vi "Parse Geometric Element with Fast Tree.vi"(8 "error in":errorcluster, 10 "Node":T1, 11 "ParseGDSII in":refnum<class "ParseGDSII.lvclass">) -> (0 "error out":errorcluster, 2 "Geometric Objects":refnum<class "Geometric.lvclass">[](array[class]), 3 "ParseGDSII out":refnum<class "ParseGDSII.lvclass">)   [LabVIEW 2019, in "ParseGDSII.lvclass"]
uses:
  ParseGDSII.lvclass
  Elements/Geometric.lvclass
  ParseGDSII.lvclass/ParseGDSII.ctl
  Fast Tree/Fast Tree.lvclass
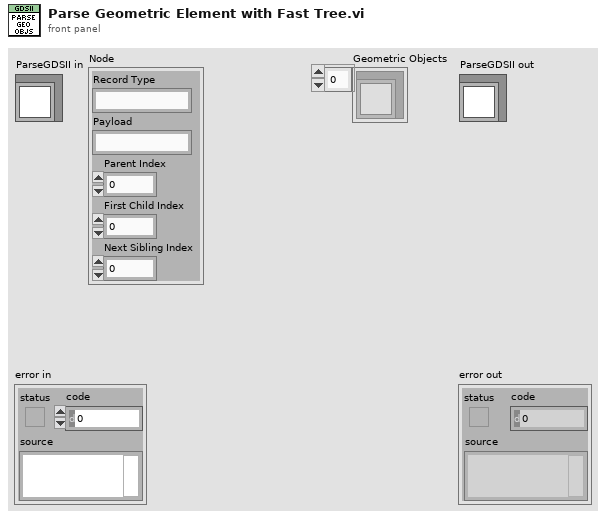
[diagram p1: front panel]
types:
  T1 = cluster{"Record Type":string, "Payload":string, "Parent Index":i32, "First Child Index":i32, "Next Sibling Index":i32}
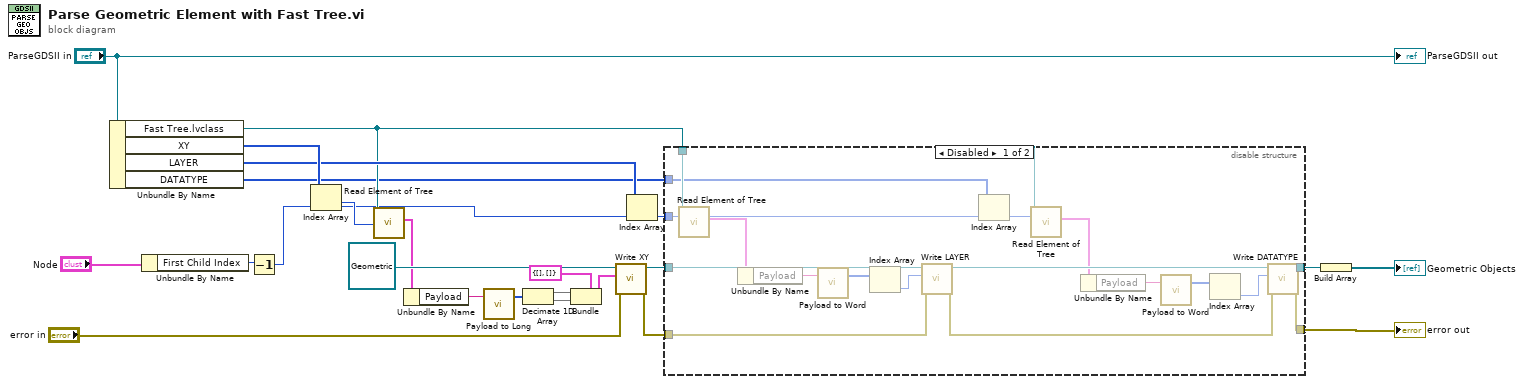
[diagram p0: block diagram]
diagram:
  n1 = Unbundle By Name("ParseGDSII in") -> ("Fast Tree.lvclass"=w3:refnum<class "Fast Tree.lvclass">, "XY"=w12:i32[], "LAYER"=w6:i32[], "DATATYPE"=w2:i32[])
  n2 = Unbundle By Name("Node") -> ("First Child Index"=w10:i32)
  n3 = Decrement(x=w10) -> (x-1=w1:i32)
  n4 = Index Array(array=w12, index=w1) -> (element=w9:i32)
  n5 = call "Read Element of Tree.vi"("index"=w9, "Fast Tree in"=w3) -> ("Node"=w8:T1)  [unwired: 7 in, 2 out]
  n6 = Unbundle By Name(w8) -> ("Payload"=w15:string)
  n7 = call "Payload to Long.vi"("Payload"=w15) -> ("Long"=w18:i32[])  [unwired: 2 in]
  n8 = Decimate 1D Array(w18) -> (w21:i32[], w20:i32[])
  n9 = Bundle(cluster=cluster{"X":i32[], "Y":i32[]} {"X"=[], "Y"=[]} ("XY"), "X"=w21, "Y"=w20) -> (w17:cluster{"X":i32[], "Y":i32[]})
  n10 = call-dynamic "Write XY.vi"("error in (no error)"="error in", "XY"=w17, "Element in"=refnum<class "Geometric.lvclass"> refnum ("Geometric")) -> ("error out"=w4:errorcluster, "Element out"=w23:refnum<class "Geometric.lvclass">)  [unwired: 7 in]
  n11 = Index Array(array=w6, index=w1) -> (element=w5:i32)
  n12 = disable-structure shown="Disabled" {
    disable-tunnel: w23 -> [w42 w45]
    disable-tunnel: [w39 w45] -> w22
    disable-tunnel: [w34 w44] -> w13
    disable-tunnel: w5 -> [w33 _]
    disable-tunnel: w4 -> [w31 w44]
    disable-tunnel: w3 -> [w28 _]
    disable-tunnel: w2 -> [w27 _]
    disable-tunnel: w1 -> [w26 _]
    frame Disabled {
      n13 = call "Read Element of Tree.vi"("index"=w33, "Fast Tree in"=w28) -> ("Node"=w32:T1)  [unwired: 7 in, 2 out]
      n14 = Unbundle By Name(w32) -> ("Payload"=w38:string)
      n15 = call "Payload to Word.vi"("Payload"=w38) -> ("Word"=w37:i16[])  [unwired: 2 in]
      n16 = Index Array(array=w37) -> (element=w43:i16)  [unwired: 1 in]
      n17 = call-dynamic "Write LAYER.vi"("error in (no error)"=w31, "LAYER"=w43, "Geometric in"=w42) -> ("error out"=w30:errorcluster, "Geometric out"=w40:refnum<class "Geometric.lvclass">)  [unwired: 7 in]
      n18 = Index Array(array=w27, index=w26) -> (element=w29:i32)
      n19 = call "Read Element of Tree.vi"("index"=w29, "Fast Tree in"=w28) -> ("Node"=w25:T1)  [unwired: 7 in, 2 out]
      n20 = Unbundle By Name(w25) -> ("Payload"=w36:string)
      n21 = call "Payload to Word.vi"("Payload"=w36) -> ("Word"=w35:i16[])  [unwired: 2 in]
      n22 = Index Array(array=w35) -> (element=w41:i16)  [unwired: 1 in]
      n23 = call-dynamic "Write DATATYPE.vi"("error in (no error)"=w30, "DATATYPE"=w41, "Geometric in"=w40) -> ("error out"=w34:errorcluster, "Geometric out"=w39:refnum<class "Geometric.lvclass">)  [unwired: 7 in]
    }
    frame Enabled {
    }
  }
  "error out" <- w13
  n24 = Build Array(w22) -> (→"Geometric Objects":refnum<class "Geometric.lvclass">[])
  "ParseGDSII out" <- "ParseGDSII in"
